vi "SendData(SubVI).vi"(8 "Error In":errorcluster, 11 "Queue in":refnum<queue>) -> (0 "Error Out":errorcluster, 3 "Queue Out":refnum<queue>)   [LabVIEW 2018]
uses:
  STM/Grafic/MOKO_Grafic_STM.ctl
  STM/Grafic/MOKO_Grafic_ITEM.ctl
  CTL/STM GRAPH.ctl
  CTL/Graph settings.ctl
  CTL/Line.ctl
  Windows/Settings/View.ctl
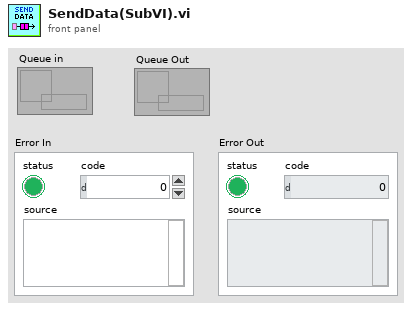
[diagram p1: front panel]
types:
  T1 = typedef "MOKO_Grafic_STM.ctl" = cluster{"main stm":T2, "STM Graph":T3}
  T2 = typedef "MOKO_Grafic_ITEM.ctl" = enum16{"idle", "init", "_____ GRAPH STATE_____ ", "Legend", "Write Graph", "Clear Graph", "close", "Screenshot", "Add Line", "Change Line", "Graph Settings", "Get Graph Appearance", "Set Graph Appearance", "Delete Line", "Autoscale", "Set Autoscale", "Hide Line", "Show Line", "Send Data", "Receive Data", "Choice Line", "_____ LED STATE_____ ", "Led Off"}
  T3 = typedef "STM GRAPH.ctl" = cluster{"Graph settings":T4, "Lines":T5[], "Data":string}
  T4 = typedef "Graph settings.ctl" = cluster{"Axis X Min":dbl, "Axis X Name":string, "Axis X Max":dbl, "Axis Y Min":dbl, " Axis Y Name":string, "Axis Y Max":dbl, "Autoscale":enum16{"Yes", "No", "Only Oy", "Only Ox"}, "Choice Line":dbl}
  T5 = typedef "Line.ctl" = cluster{"Width":dbl, "Color":i64, "Array Oy":dbl[], "Array Ox":dbl[], "Name":string, "Plot Visible":T6}
  T6 = typedef "View.ctl" = bool
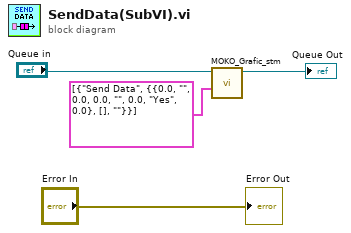
[diagram p0: block diagram]
diagram:
  n1 = call "MOKO_Grafic_stm.vi"("StateMachineSteps"=T1[] [{"main stm"=enum."Send Data", "STM Graph"={"Graph settings"={"Axis X Min"=0.0, "Axis X Name"="", "Axis X Max"=0.0, "Axis Y Min"=0.0, " Axis Y Name"="", "Axis Y Max"=0.0, "Autoscale"=enum."Yes", "Choice Line"=0.0}, "Lines"=[], "Data"=""}}], "queue in"="Queue in") -> ("queue out"=→"Queue Out":refnum<queue>)  [unwired: 8 in, 1 out]
  "Error Out" <- "Error In"
